vi "mqttServer.vi"() -> ()   [LabVIEW 2019]
uses:
  <vilib>/LabVIEW Open Source Project/MQTT Connection/MQTT_Base/Base Class/MQTT_Base.lvclass/MQTT_Base.ctl
  <vilib>/G Open Source Project for LabVIEW/MQTT Broker/Server class/Server.lvclass/Server.ctl
  <vilib>/LabVIEW Open Source Project/MQTT Control Packets/Control Packets/PUBLISH/PUBLISH.lvclass
  C:/Program Files (x86)/National Instruments/LabVIEW 2019/vi.lib/LabVIEW Open Source Project/MQTT Control Packets/Control Packets/ControlPacket/ControlPacket.lvclass
  <vilib>/LabVIEW Open Source Project/MQTT Control Packets/Control Packets/ControlPacket/ControlPacket.lvclass/ControlPacket.ctl
  <vilib>/LabVIEW Open Source Project/MQTT TCP Connection/MQTT_TCP/Connection/TCPConnection.lvclass
  C:/Program Files (x86)/National Instruments/LabVIEW 2019/vi.lib/LabVIEW Open Source Project/MQTT Connection/MQTT_Connection/Connection/Connection.lvclass
  <vilib>/G Open Source Project for LabVIEW/MQTT Broker/Server class/Server.lvclass
  C:/Program Files (x86)/National Instruments/LabVIEW 2019/vi.lib/LabVIEW Open Source Project/MQTT Connection/MQTT_Base/Base Class/MQTT_Base.lvclass
  <vilib>/LabVIEW Open Source Project/Epoch Date & Time/epoch.UNIX/Epoch.UNIX.lvclass
  C:/Program Files (x86)/National Instruments/LabVIEW 2019/vi.lib/LabVIEW Open Source Project/Epoch Date & Time/epoch/Epoch.lvclass
  <vilib>/LabVIEW Open Source Project/Epoch Date & Time/Get Epoch Time.vi
  <vilib>/LabVIEW Open Source Project/MQTT Connection/MQTT_Base/Base Class/MQTT_Base.lvclass
panel:
  in  "Trace Messages":bool
  out "Error Server":errorcluster
  out "NbConnections":u32
  out "Inbound Log":string
  in  "AutoScroll":bool=TRUE
  in  "Clear Log":bool
  # "Native LabVIEW MQTT Broker"
  # "G Open Source Project for LabVIEW\nhttps://github.com/LabVIEW-Open-Source/LV-MQTT-Broker"
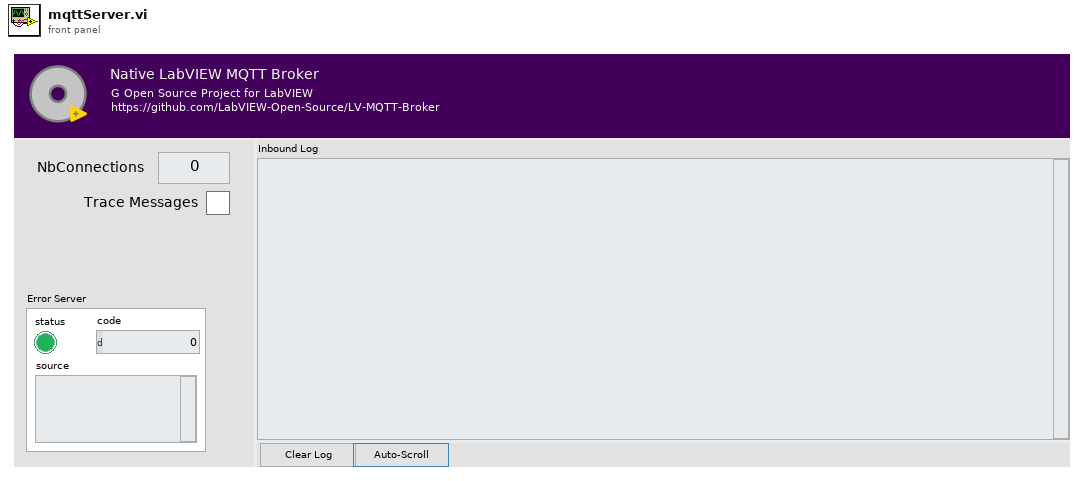
[diagram p1: front panel]
types:
  T1 = typedef "MQTT Base.lvlib/MQTT_Base.lvclass/Public Events -- cluster.ctl" = cluster{"Stop Event":refnum<user-event>, "Error Event":refnum<user-event>, "Inbound Message":refnum<user-event>}
  T2 = typedef "MQTT Server.lvlib/Server.lvclass/Public Events -- cluster.ctl" = cluster{"NbConnections":refnum<user-event>}
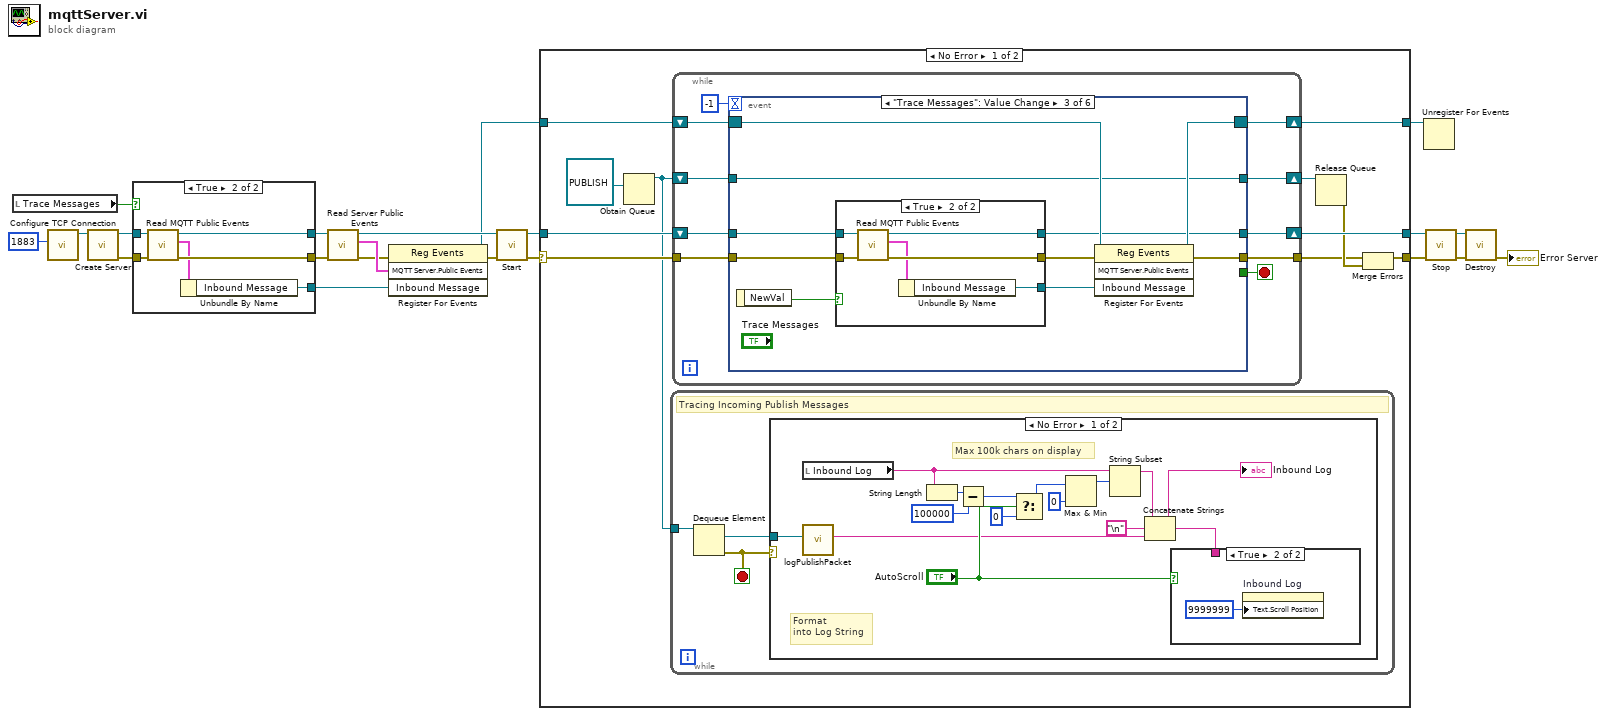
[diagram p0: block diagram]
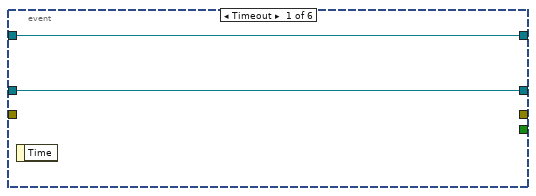
[diagram p5: hidden frame]
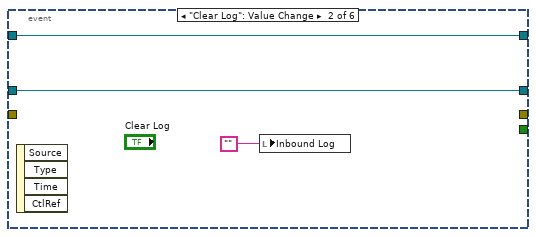
[diagram p6: hidden frame]
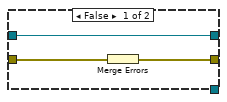
[diagram p7: hidden frame]
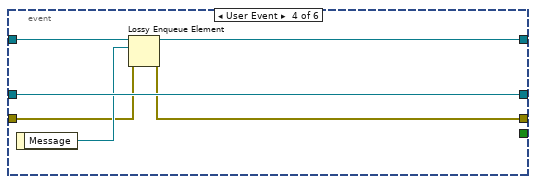
[diagram p8: hidden frame]
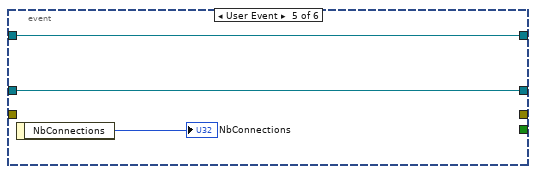
[diagram p9: hidden frame]
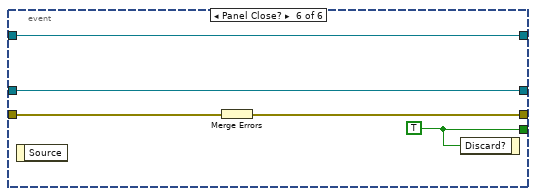
[diagram p10: hidden frame]
diagram:
  n1 = local read "Trace Messages"() -> (w1:bool)
  n2 = call <vilib>:"Configure TCP Connection.vi"("remote port (80)"=u16 1883) -> ("TCPConnection"=w7:refnum<class "TCPConnection.lvclass">)  [unwired: 9 in, 1 out]
  n3 = call <vilib>:"Create Server.vi"("Connection Configuration"=w7) -> ("error out"=w6:errorcluster, "Server"=w4:refnum<class "Server.lvclass">)  [unwired: 9 in]
  n4 = case shown="True" w1 {
    tunnel: w6 -> [w22 w29]
    tunnel: [w22 w28] -> w5
    tunnel: w4 -> [w23 w27]
    tunnel: [w23 w26] -> w3
    tunnel: [_ w24] -> w2
    frame False {
    }
    frame True {
      n5 = call <vilib>:"Read MQTT Public Events.vi"("error in (no error)"=w29, "MQTT_Base in"=w27) -> ("error out"=w28:errorcluster, "MQTT Public Events"=w25:T1, "MQTT_Base out"=w26:refnum<class "Server.lvclass">)  [unwired: 7 in]
      n6 = Unbundle By Name(w25) -> ("Inbound Message"=w24:refnum<user-event>)
    }
  }
  n7 = call <vilib>:"Read Server Public Events.vi"("error in (no error)"=w5, "Server in"=w3) -> ("error out"=w9:errorcluster, "MQTT Server.Public Events"=w10:T2, "Server out"=w13:refnum<class "Server.lvclass">)  [unwired: 7 in]
  n8 = register-events(error in=w9, w10, w2) -> (reference out=w11:refnum<event-registration>, error out=w15:errorcluster)  [unwired: 1 in]
  n9 = call <vilib>:"Start.vi"("error in (no error)"=w15, "MQTT_Base in"=w13) -> ("error out"=w16:errorcluster, "MQTT_Base out"=w14:refnum<class "Server.lvclass">)  [unwired: 7 in, 1 out]
  n10 = case shown="No Error" w16 {
    selector: w16 -> [w36 w107]
    tunnel: w14 -> [w40 w109]
    tunnel: [w39 w109] -> w19
    tunnel: w11 -> [w38 w108]
    tunnel: [w37 w108] -> w12
    tunnel: [w32 w107] -> w21
    frame No Error {
      n11 = Obtain Queue(element data type=refnum<class "PUBLISH.lvclass"> refnum ("Message")) -> (queue out=w31:refnum<queue>)  [unwired: 4 in, 2 out]
      n12 = while {
        tunnel: w31 -> [w43]
        stop <- w42 stop-if-true
        # "Tracing Incoming Publish Messages"
        n13 = Dequeue Element(queue=w43) -> (element=w41:refnum<class "PUBLISH.lvclass">, error out=w42:errorcluster)  [unwired: 2 in, 2 out]
        n14 = case shown="No Error" w42 {
          tunnel: w41 -> [w45 _]
          frame No Error {
            # "Max 100k chars on display"
            # "Format\ninto Log String"
            n15 = local read "Inbound Log"() -> (w56:string)
            n16 = call "logPublishPacket.vi"("PUBLISH packet"=w45) -> ("Publish Log"=w46:string)  [unwired: 10 in]
            n17 = String Length(string=w56) -> (length=w55:i32)
            n18 = Subtract(x=w55, y=100000 ("length (rest)")) -> (x-y=w50:i32)
            n19 = Select(t=w50, s="AutoScroll", f=0 ("y")) -> (s? t:f=w49:i32)
            n20 = Max & Min(x=w49, y=0) -> (max(x,y)=w53:i32)  [unwired: 1 out]
            n21 = String Subset(string=w56, offset (0)=w53) -> (substring=w52:string)  [unwired: 1 in]
            n22 = Concatenate Strings(w52, "\n", w46) -> (w44:string)
            "Inbound Log" <- w44
            n23 = case shown="True" "AutoScroll" {
              tunnel: w44 -> [_ _]
              frame False {
              }
              frame True {
                n24 = property on="Inbound Log" class="Str"("Text.Scroll Position"=u32 9999999) -> ()  [unwired: 2 in, 2 out]
              }
            }
          }
          frame Error {
          }
        }
      }
      n25 = while {
        shift-right: [w65] -> w39
        shift-left: w40 -> [w67]
        tunnel: [w62] -> w33
        tunnel: w36 -> [w61]
        shift-right: [w63] -> w37
        shift-left: w38 -> [w64]
        shift-right: [w59] -> w35
        shift-left: w31 -> [w60]
        stop <- w66 stop-if-true
        n26 = event shown="[2] \"Trace Messages\": Value Change" {
          selector: w64 -> [_ _ w83 _ _ _]
          dyn-events: [_ _ w82 _ _ _] -> w63
          timeout: -1 -> [_ _ _ _ _ _]
          tunnel: w67 -> [w70 w73 w79 w98 w101 w106]
          tunnel: [_ _ _ _ _ w105] -> w66
          tunnel: [w70 w73 w80 w98 w101 w106] -> w65
          tunnel: [_ _ w81 _ _ w103] -> w62
          tunnel: w61 -> [_ _ w77 w93 _ w104]
          tunnel: [_ _ _ w94 _ _] -> _
          tunnel: w60 -> [w69 w72 w74 w97 w99 w102]
          tunnel: [w69 w72 w74 w95 w99 w102] -> w59
          event Timeout {
            n27 = event-data() -> ()  [unwired: 1 in, 1 out]
          }
          event "Clear Log": Value Change {
            n28 = event-data() -> ()  [unwired: 1 in, 4 out]
            n29 = local write "Inbound Log"("") -> ()
          }
          event "Trace Messages": Value Change {
            n30 = event-data() -> ("NewVal"=w75:bool)  [unwired: 1 in]
            n31 = case shown="True" w75 {
              tunnel: [w86 w92] -> w80
              tunnel: w79 -> [w86 w91]
              tunnel: [w85 w90] -> w78
              tunnel: w77 -> [w84 w89]
              tunnel: [_ w88] -> w76
              frame False {
                n32 = Merge Errors(w84) -> (w85:errorcluster)
              }
              frame True {
                n33 = call <vilib>:"Read MQTT Public Events.vi"("error in (no error)"=w89, "MQTT_Base in"=w91) -> ("error out"=w90:errorcluster, "MQTT Public Events"=w87:T1, "MQTT_Base out"=w92:refnum<class "Server.lvclass">)  [unwired: 7 in]
                n34 = Unbundle By Name(w87) -> ("Inbound Message"=w88:refnum<user-event>)
              }
            }
            n35 = register-events(reference=w83, error in=w78, w76) -> (reference out=w82:refnum<event-registration>, error out=w81:errorcluster)  [unwired: 1 in]
          }
          event User Event {
            n36 = event-data() -> ("Message"=w96:refnum<class "PUBLISH.lvclass">)  [unwired: 1 in]
            n37 = Lossy Enqueue Element(queue=w97, element=w96, error in (no error)=w93) -> (queue out=w95:refnum<queue>, error out=w94:errorcluster)  [unwired: 2 out]
          }
          event User Event {
            n38 = event-data() -> ("NbConnections"=→"NbConnections":u32)  [unwired: 1 in]
          }
          event Panel Close? {
            w105 = TRUE ("Discard?")
            n39 = event-data() -> ()  [unwired: 1 in, 1 out]
            n40 = Merge Errors(w104) -> (w103:errorcluster)
            n41 = event-data("Discard?"=w105) -> ()  [unwired: 1 in, 1 out]
          }
        }
      }
      n42 = Release Queue(queue=w35) -> (error out=w34:errorcluster)  [unwired: 2 in, 2 out]
      n43 = Merge Errors(w33, w34) -> (w32:errorcluster)
    }
    frame Error {
    }
  }
  n44 = Unregister For Events(event registration refnum=w12) -> ()  [unwired: 1 in, 1 out]
  n45 = call <vilib>:"Stop.vi"("error in (no error)"=w21, "MQTT_Base in"=w19) -> ("error out"=w20:errorcluster, "MQTT_Base out"=w18:refnum<class "Server.lvclass">)  [unwired: 7 in, 1 out]
  n46 = call <vilib>:"Destroy.vi"("error in (no error)"=w20, "MQTT_Base in"=w18) -> ("error out"=→"Error Server":errorcluster)  [unwired: 8 in, 1 out]
